vi "_CSMOFGV TagMap.vi"(8 "error in (no error)":errorcluster, 9 "Wait (5000 ms)":i32, 11 "CSM Name":string) -> (0 "error out":errorcluster, 1 "Waited (ms)":u32, 3 "TagMap":refnum<data-value>)   [LabVIEW 2017, in "Communicable State Machine.lvlib"]
uses:
  Communicable State Machine.lvlib
  _CSMOFGVOPER.ctl
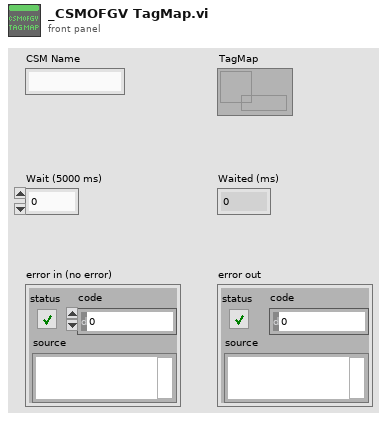
[diagram p1: front panel]
types:
  T1 = typedef "Communicable State Machine.lvlib/_CSMOFGVOPER.ctl" = enum16{"Create If not Exist", "Get By Name", "List", "Check If Name Exists", "Release", "Module Status", "Create Status Event Handler", "Destroy Status Event Handler", "Clear Invalid Objs"}
  T2 = typedef "Communicable State Machine.lvlib/_CSMObj.ctl" = cluster{"info":T3, "Refs":T5}
  T3 = typedef "Communicable State Machine.lvlib/_CSMObj-Info.ctl" = cluster{"Module Name":string, "Requested Name":string, "Group Name":string, "Mode":T4, "Allowed Messages":string[]}
  T4 = typedef "Communicable State Machine.lvlib/_CSM_MODE.ctl" = enum16{"Not Exist", "Stand Alone", "CSM", "Worker", "Worker Agent", "Chain Node", "Chain"}
  T5 = typedef "Communicable State Machine.lvlib/_CSMObj-Refs.ctl" = cluster{"WatchDogQ":refnum<queue>, "CSMDataDVR":refnum<data-value>, "Queue":T6, "GroupDataDVR":refnum<data-value>, "TagMap":refnum<data-value>, "ExitEvent":refnum<user-event>, "NewStateEvent":refnum<user-event>, "StatusChangeEvent":refnum<user-event>}
  T6 = typedef "Communicable State Machine.lvlib/Priority Queue.ctl" = cluster{"HPriorityQ":refnum<queue>, "LowPriorityQ":refnum<queue>}
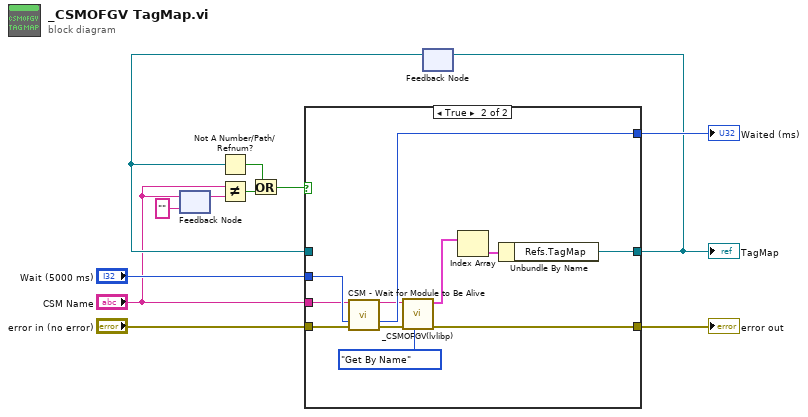
[diagram p0: block diagram]
diagram:
  n1 = feedback #1("" ("CSM Name")) -> (w2:string)
  n2 = feedback-in #1("CSM Name") -> ()
  n3 = Not Equal?(x="CSM Name", y=w2) -> (x != y?=w6:bool)
  n4 = feedback #2() -> (w7:refnum<data-value>)  [unwired: 1 in]
  n5 = Not A Number/Path/Refnum?(number/path/refnum=w7) -> (NaN/Path/Refnum?=w5:bool)
  n6 = Or(x=w5, y=w6) -> (x .or. y?=w4:bool)
  n7 = case shown="True" w4 {
    tunnel: "Wait (5000 ms)" -> [_ w25]
    tunnel: [_ w24] -> w11
    tunnel: "CSM Name" -> [_ w22]
    tunnel: [w13 w17] -> w10
    tunnel: "error in (no error)" -> [w13 w16]
    tunnel: [w14 w15] -> w8
    tunnel: w7 -> [w14 _]
    frame False {
    }
    frame True {
      n8 = call "CSM - Wait for Module to Be Alive.vi"("CSM Name"=w22, "Wait (5000 ms)"=w25, "error in (no error)"=w16) -> ("CSM Name (Dup)"=w23:string, "Waited (ms)"=w24:u32, "error out"=w21:errorcluster)  [unwired: 10 in]
      n9 = call "_CSMOFGV(lvlibp).vi"("Operation"=_CSMOFGVOPER."Get By Name", "Error In"=w21, "Name (\"\" to Use UUID) In"=w23) -> ("error out"=w17:errorcluster, "Array"=w19:T2[])  [unwired: 6 in, 1 out]
      n10 = Index Array(array=w19) -> (element=w20:T2)  [unwired: 1 in]
      n11 = Unbundle By Name(w20) -> ("Refs.TagMap"=w15:refnum<data-value>)
    }
  }
  "Waited (ms)" <- w11
  "TagMap" <- w8
  "error out" <- w10
  n12 = feedback-in #2(w8) -> ()
